vi "setExposureTime.vi"(0 "CCD in":refnum<class "CCD.lvclass">, 1 "exposure time":i32, 5 "error in (no error)":errorcluster) -> (14 "CCD out":refnum<class "CCD.lvclass">, 15 "results-JSON string":string, 16 "ID":i32, 17 "returned command":string, 18 "error string (if existing)":string, 19 "error out":errorcluster)   [LabVIEW 2023, in "CCD.lvclass"]
uses:
  CCD.lvclass
  CCD.lvclass/CCD.ctl
  20f7d3bd-08ac-4524-9bed-df36c1da25a0.vi
  GenericDevice/GenericDevice.lvclass
  f686cde6-bd46-49cb-aabb-d3acb6fd99c9.vi
panel:
  # "Connector Pane"
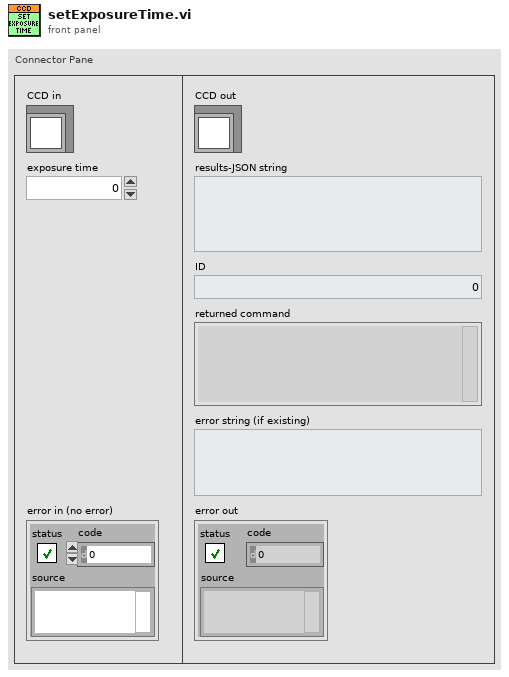
[diagram p1: front panel]
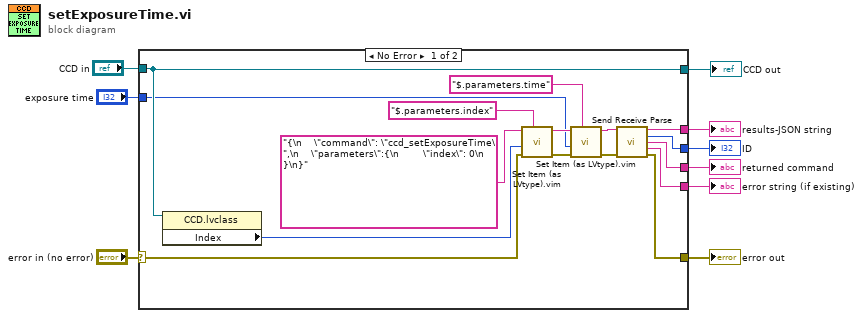
[diagram p0: block diagram]
diagram:
  n1 = case shown="No Error" "error in (no error)" {
    selector: "error in (no error)" -> [w21 w27]
    tunnel: [w13 w27] -> w8
    tunnel: [w23 w26] -> w6
    tunnel: "CCD in" -> [w23 w26]
    tunnel: [w14 _] -> w1
    tunnel: "exposure time" -> [w15 _]
    tunnel: [w12 _] -> w4
    tunnel: [w11 _] -> w3
    tunnel: [w10 _] -> w2
    frame No Error {
      n2 = property class="CCD.lvclass"(reference=w23) -> ("Index"=w22:i32)  [unwired: 1 in, 2 out]
      n3 = call "Set Item (as LVtype).vim"("$Path or Item Name"="$.parameters.index", "error in (no error)"=w21, "Anything"=w22, "JSON"="{\n    \"command\": \"ccd_setExposureTime\",\n    \"parameters\":{\n        \"index\": 0\n    }\n}") -> ("error out"=w18:errorcluster, "<JSON>"=w20:string)  [unwired: 4 in, 1 out]
      n4 = call "Set Item (as LVtype).vim"("$Path or Item Name"="$.parameters.time", "error in (no error)"=w18, "Anything"=w15, "JSON"=w20) -> ("error out"=w17:errorcluster, "<JSON>"=w19:string)  [unwired: 4 in, 1 out]
      n5 = call "Send Receive Parse.vi"("<JSON>"=w19, "error in"=w17) -> ("results-JSON string"=w14:string, "ID"=w12:i32, "returned command"=w11:string, "error string (if existing)"=w10:string, "error out"=w13:errorcluster)  [unwired: 9 in]
    }
    frame Error {
    }
  }
  "error out" <- w8
  "CCD out" <- w6
  "ID" <- w4
  "returned command" <- w3
  "error string (if existing)" <- w2
  "results-JSON string" <- w1
